vi "AlliGator Get Control Notebook String.vi"(8 "error in (no error)":errorcluster, 9 "Value":variant, 11 "Control Label":string) -> (0 "error out":errorcluster, 3 "Notebook String":string)   [LabVIEW 2021, in "AlliGator Settings.lvlib"]
doc: "Formats the input <B>Value</B> of the control whose <B>Control Label</b> is provided into a string.\n\nA special case is needed when units are involved, otherwise the default case should be able to handle all other cases."
uses:
  AlliGator Settings.lvlib
  Graphs/XY Graph/XY Graph Plot Shift Method.ctl
  AlliGator Settings List.ctl
  Decay Analysis/Decay Preprocessing/AlliGator Baseline Subtraction Method.ctl
  Phasor/Phasor Calibration Type.ctl
  Phasor Calibration/AlliGator Calibration Map Algorithm.ctl
  Phasor/Phasor Explorer Decay Parameters.ctl
  Phasor/Phasor IRF Model.ctl
  Graphs/XY Graph/XY Graph Plot Shift Parameters.ctl
  AlliGator Define Gates to.ctl
  Phasor/Phasor Explorer Display Parameters.ctl
  Phasor/Phasor Type of Series.ctl
  Fits/IRF(X)PSED/Decay Fit Parameters & Derived Quantities List v2.ctl
  Decay Analysis/Decay Fit/AlliGator Decay Fit Parameter Constraints 2.ctl
  Fits/IRF(X)PSED/Decay Fit Parameters In List.ctl
  Phasor/Phasor Explorer Gate Parameters.ctl
  Phasor/Phasor Gate Type.ctl
  Phasor/Phasor Type of User-defined Function.ctl
  AlliGator Gate Arithmetic.ctl
  AlliGator Gates to Keep.ctl
  Fits/IRF(X)PSED/MLE Baseline Offset Type.ctl
  AlliGator Background Subtraction Parameters.ctl
  SwissSPAD/SwissSPAD Live_Image Display Options.ctl
  Phasor/Phasor Ratio Type.ctl
  AlliGator High Count Pixels Rejection Options.ctl
  Fits/IRF(X)PSED/IRF(X)PSED Extraction Options.ctl
  Fits/IRF(X)PSED/Fourier Series Smoothing Option.ctl
  Fits/IRF(X)PSED/Fourier Series Truncation.ctl
  Fits/IRF(X)PSED/IRF Extraction Method.ctl
  Arrays/Kernel Type.ctl
  AlliGator Low Count Pixels Rejection Options.ctl
  Phasor/Phasor Explorer Phasor Parameters.ctl
  Phasor/Phasor Calculation Type.ctl
  Phasor/Phasor SEPL Type.ctl
  Phasor Plot/AlliGator Phasor Plot Size.ctl
  Phasor Ratio/AlliGator Phasor Ratio Color-Coded Quantity.ctl
  Phasor/Pseudo UC Additional Parameters.ctl
  AlliGator Python Settings.ctl
  Image/Image Save File Format.ctl
  Fits/Square Pulse/Square Pulse Options.ctl
  Fits/Square Pulse/Square Pulse Levels Type.ctl
  Graphs/XY Graph/XY Graph Plot Data.ctl
  Math/Advanced Signal Processing Toolkit/Wavelet Analysis Options.ctl
  Variant/Variant to Data/Variant to U32.vi
  Variant/Variant to Data/Variant to I32.vi
  Variant/Variant to Data/Variant to String.vi
  Variant/Variant to Data/Variant to Boolean.vi
  Variant/Variant to Data/Variant to DBL.vi
  Variant/Variant to Data/Variant to Path.vi
  Variant/Variant to Data/Variant to [String].vi
  Variant/Variant to Data/Variant to U16.vi
  Variant/Variant to Data/Variant to [DBL].vi
  Variant/Variant to Data/Variant to Data.lvlib
  Phasor Plot/AlliGator Phasor Plot.lvlib
  Graphs/XY Graph/XY Graph Add-Ons.lvlib
  Image/Image.lvlib
  Decay Analysis/Decay Preprocessing/AlliGator Decay Preprocessing.lvlib
  Fits/Fits.lvlib
  Decay Analysis/Decay Fit/AlliGator Decay Fit.lvlib
  Phasor/Phasor.lvlib
  Strings/Strings.lvlib
  Arrays/Arrays.lvlib
  Math/Math.lvlib
  Phasor/Phasor Explorer.lvlib
  Phasor Ratio/AlliGator Phasor Ratio.lvlib
  Phasor Calibration/AlliGator Phasor Calibration.lvlib
  SwissSPAD/SwissSPAD Live.lvlib
  Variant/Variant.lvlib
panel:
  in  "Type":T1
  # "see the AlliGator License on the block diagram (Ctrl+E or Window:Show Block Diagram)"
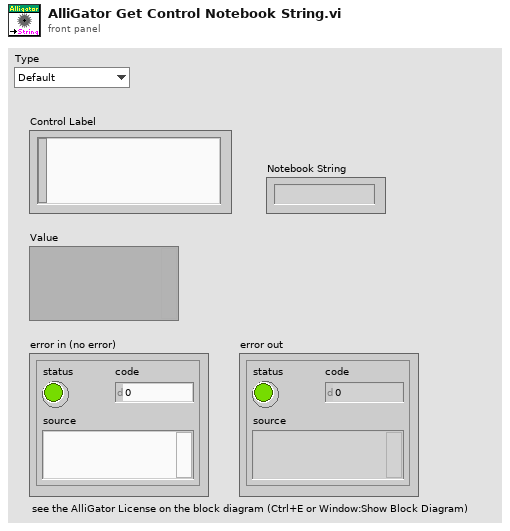
[diagram p1: front panel]
types:
  T1 = typedef "XY Graph Add-Ons.lvlib/XY Graph Plot Shift Method.ctl" = enum16{"Default", "CFD", "Threshold", "Cross-Correlation"}
  T2 = typedef "AlliGator Settings.lvlib/AlliGator Settings List.ctl" = enum16{"GUI:Visible Settings Tab", "GUI:Last Run Version", "Source Image:Use Image Histogram for Contrast", "Source Image:Low Count Pixels Rejection Options", "Source Image:High Count Pixels Rejection Options", "Source Image:Use Image Brightness", "Source Image:Blend Overlay with Image Background", "Source Image:Use Fixed ROI Diameter", "Source Image:ROI Diameter", "Source Image:ROI Center Color", "Source Image:Peak Threshold", "Source Image:Intensity Threshold", "Source Image:Image Binning Options", "Source Image:Image Smoothing Options", "Source Image:Image Histogram Active", "Source Image:Invert Binary Mask", "Source Image:Hot Pixel Removal", "Source Image:Overlay Analyzed ROI Center", "Source Image:Auto-Adjust Contrast", "Source Image:Histogram Lower Percentile", "Source Image:Histogram Upper Percentile", "Source Image:Save Source Image", "Source Image:Scale Bar Options", "Source Image:Image Resolution (Pixel Size)", "Source Image:Flatfield Correction", "Source Image:Show Dead Left Columns Correction", "Source Image:Dead Left Columns Correction", "Source Image:Image Pre-Processing Operations Order", "Source Image:Overlay ROI Median", "Source Image:Median Overlay Color", "Data Information:Gate Width", "Data Information:Nanotime Gate Separation", "Data Information:Macrotime Gate Separation", "Data Information:Gate Step", "Data Information:# Gates", "Data Information:Gate Image Exposure", "Data Information:Gate Image Integration", "Data Information:Gates to Skip", "Data Information:Gates to Keep", "Data Information:Define Gates to", "Data Information:Channel Name", "Data Information:Available Channel Names", "Data Information:Channel Arithmetic", "Data Information:Background File Subtraction", "Data Information:Background File", "Data Information:Background Scaling Factor", "Data Information:Background Pile-up Correction", "Data Information:Background Pixel Well Capacity", "Data Information:Laser Period", "Data Information:SYNC Period", "Data Information:Pile-up Correction", "Data Information:Pixel Well Capacity", "Data Information:Dataset Scaling Factor", "Fluorescence Decay_Decay Pre-Processing:Reverse Gates", "Fluorescence Decay_Decay Pre-Processing:Verbose Decay Pre-Processing", "Fluorescence Decay_Decay Pre-Processing:Use Decay Pre-Processing", "Fluorescence Decay_Decay Pre-Processing:Background Subtraction", "Fluorescence Decay_Decay Pre-Processing:Background Definition Range", "Fluorescence Decay_Decay Pre-Processing:Baseline Subtraction Method", "Fluorescence Decay_Decay Pre-Processing:Decay Pre-Processing Operations Order", "Fluorescence Decay_Decay Pre-Processing:Smoothing Parameter", "Fluorescence Decay_Decay Pre-Processing:Shift Decay", "Fluorescence Decay_Decay Pre-Processing:Decay Shift Parameters", "Fluorescence Decay_Decay Pre-Processing:Fold Decay", "Fluorescence Decay_Decay Pre-Processing:# Folds", "Fluorescence Decay_Decay Pre-Processing:1-Normalize Decay", "Fluorescence Decay_Decay Pre-Processing:[0-1]-Normalize Decay", "Fluorescence Decay_Decay Pre-Processing:Smoothen Decay", "Fluorescence Decay_Decay Pre-Processing:Extrapolate Decay", "Fluorescence Decay_Decay Pre-Processing:Use Periodicity", "Fluorescence Decay_Decay Pre-Processing:Use Cursors", "Fluorescence Decay_Decay Pre-Processing:Tail Fraction", "Fluorescence Decay_Decay Pre-Processing:Head Fraction", "Fluorescence Decay_Decay Pre-Processing:Additional Points", "Fluorescence Decay_Decay Pre-Processing:Straighten Decay", "Fluorescence Decay_Decay Pre-Processing:Constant Background", "Fluorescence Decay_Decay Pre-Processing:Pixel-Normalize Decay", "Fluorescence Decay_Advanced Analysis:Extract IRF instead of Decay", "Fluorescence Decay_Advanced Analysis:IRF Extraction Options", "Fluorescence Decay_Advanced Analysis:IRF Optimization Options", "Fluorescence Decay_Advanced Analysis:Square Pulse Options", "Fluorescence Decay_Advanced Analysis:IRF Order", "Fluorescence Decay_Advanced Analysis:IRF Time Constants", "Fluorescence Decay_Advanced Analysis:Wavelet Analysis Options", "Fluorescence Decay_Advanced Analysis:Average Lifetime Options", "Fluorescence Decay_Fit Options:Fit Options", "Fluorescence Decay_Fit Options:Use Legacy Fitting Approach", "Fluorescence Decay_Fit Options:Use Data Information Laser Period", "Fluorescence Decay_Fit Parameters:Displayed Fit Parameters", "Fluorescence Decay_Fit Parameters:Fit Parameter Constraints", "Fluorescence Decay_Fit Parameters:Export Tabulated Results", "Fluorescence Decay_Fit Parameters:MLE Baseline Offset Type", "Fluorescence Decay_Fit Parameters:MLE Baseline Offset", "Fluorescence Decay_Fit Parameters:Guess Parameter Names", "Fluorescence Decay_Fit Parameters:Guess Parameter Values", "Fluorescence Decay_Fit Parameters:Guess Parameters Options", "Fluorescence Decay_Fit Parameters:Optimal Offset Selection Criterion", "Fluorescence Decay_Styles:Show Last Decay Only", "Fluorescence Decay_Styles:Decay Graph Color Array", "Fluorescence Decay:Decay Graph Active", "Fluorescence Decay Statistics:Min Peak Value", "Fluorescence Decay Statistics:Reject Low Decay Peak Pixels", "Fluorescence Decay Statistics:Reject High Decay Peak Pixels", "Fluorescence Decay Statistics:Max Peak Value", "Time Traces:Use File Timestamp", "Time Traces:Time Step", "Time Traces:Use Intensity Correction File", "Time Traces:Intensity Correction File", "Phasor Plot:Phasor Plot Smoothing Options", "Phasor Plot:Phasor Plot Size", "Phasor Plot:Phasor Plot Graphics Options", "Phasor Plot:Cumulative Phasor Plot", "Phasor Plot:Use Phasor Brightness", "Phasor Plot:Blend Overlay with Phasor Background", "Phasor Plot:Save Phasor Plot", "Phasor Plot:Show References", "Phasor Plot:Phasor Ratio Decay Range", "Phasor Plot:Exponential Fading", "Phasor Plot:Phasor Ratio Reference Colors", "Phasor Plot:Reference Radius", "Phasor Plot:Show Color Map Vertices", "Phasor Plot:Phasor Plot Active", "Phasor Plot:Phasor Ratio Color Map Type", "Phasor Plot:Phasor Ratio Color Map", "Phasor Plot:Phasor Ratio Display Range", "Phasor Plot:Selected Image ROI(s)", "Phasor Plot:All Image ROIs", "Phasor Plot:Selected Phasor Plot ROI(s)", "Phasor Plot:All Phasor Plot ROIs", "Phasor Plot:Phasor Ratio Color-Coded Quantity", "Phasor Plot:Store Phasor Harmonics", "Phasor Plot:Draw Reference Segment", "Phasor Plot:User-Defined Quantity", "Phasor Plot:Color Scale High Color", "Phasor Plot:Color Scale Low Color", "Phasor Graph:Phasor Frequency", "Phasor Graph:Phasor Ratio Type", "Phasor Graph:Pixel-level Phasor Computation", "Phasor Graph:Save Phasor Graph", "Phasor Graph:Phasor Graph Active", "Phasor Graph:Phasor SDV Options", "Phasor Calibration:Use Backup Calibration if needed", "Phasor Graph:Define Shortest Lifetime as", "Phasor Calibration:Backup Calibration Type", "Phasor Calibration:Calibration Type", "Phasor Calibration:Calibration Lifetime", "Phasor Calibration:Calibration Map Algorithm", "Single-Exponential Phasor Locus (SEPL):Gate Parameters", "Single-Exponential Phasor Locus (SEPL):User-defined Gate", "Single-Exponential Phasor Locus (SEPL):User-defined IRF", "Single-Exponential Phasor Locus (SEPL):Phasor Parameters", "Single-Exponential Phasor Locus (SEPL):Decay & IRF Parameters", "Single-Exponential Phasor Locus (SEPL):Display Parameters", "Lifetime Analysis:Decay Analysis Parameters", "Lifetime Analysis:Lifetime Map Active", "Plugins:Python Settings", "Miscellaneous:Verbose Mode", "Miscellaneous:Beep after Script", "Miscellaneous:Saved Image File Format", "Miscellaneous:Exported Gate Image Settings", "Miscellaneous:Include Loading in Timing", "Miscellaneous:Verbose Settings Mode", "Miscellaneous:Histogram Options", "Miscellaneous:Beep on Error", "Miscellaneous:# Logical Processors Used", "Miscellaneous:ROI Description Max Characters", "Miscellaneous:Verbose Error Mode", "Miscellaneous:Transparent Mask Color"}
  T3 = cluster{"Min Gate":dbl[unit], "Max Gate":dbl[unit]}
  T4 = enum16{"Single Calibration", "Nearest Valid Calibration"}
  T5 = typedef "AlliGator Decay Preprocessing.lvlib/AlliGator Baseline Subtraction Method.ctl" = enum16{"Mean", "Min", "Square Gated Single-Exponential", "File", "Constant"}
  T6 = typedef "Phasor.lvlib/Phasor Calibration Type.ctl" = enum16{"None", "Single Phasor", "Phasor Series", "Phasor Map"}
  T7 = typedef "AlliGator Phasor Calibration.lvlib/AlliGator Calibration Map Algorithm.ctl" = enum16{"Simple Search", "Min Distance"}
  T8 = typedef "Phasor Explorer.lvlib/Phasor Explorer Decay Parameters.ctl" = cluster{"Lifetime":dbl[unit], "IRF Offset":dbl[unit], "IRF Period":dbl[unit], "Normalized Decays":bool, "IRF Model":T9, "IRF Parameter 1":dbl[unit]}
  T9 = typedef "Phasor.lvlib/Phasor IRF Model.ctl" = enum16{"Dirac", "Exponential"}
  T10 = typedef "XY Graph Add-Ons.lvlib/XY Graph Plot Shift Parameters.ctl" = cluster{"Type":T1, "Shift":dbl[unit], "Threshold":dbl, "Rotate":bool}
  T11 = typedef "AlliGator Settings.lvlib/AlliGator Define Gates to.ctl" = enum32{"Skip", "Keep"}
  T12 = typedef "Phasor Explorer.lvlib/Phasor Explorer Display Parameters.ctl" = cluster{"# Points":i32, "Ramp Type":enum16{"Linear", "Logarithmic"}, "Type of Series":T13, "Min tau":dbl[unit], "Max tau":dbl[unit], "Include 0":bool, "Include Infinity":bool}
  T13 = typedef "Phasor.lvlib/Phasor Type of Series.ctl" = enum16{"1-Exp Decays", "Linear Combination of 1-Exp"}
  T14 = typedef "AlliGator Decay Fit.lvlib/AlliGator Decay Fit Parameter Constraints 2.ctl" = cluster{"Fit Parameter":T15, "Min Value":dbl, "Max Value":dbl, "Global":bool, "Used":bool}
  T15 = typedef "Fits.lvlib/Decay Fit Parameters In List.ctl" = enum16{"Offset", "Baseline", "A_1", "tau_1", "A_2", "tau_2"}
  T16 = typedef "Phasor Explorer.lvlib/Phasor Explorer Gate Parameters.ctl" = cluster{"First Gate Start":dbl[unit], "Use Gate Center":bool, "Gate Width":dbl[unit], "Gate Step":dbl[unit], "# Gates":dbl, "Gate Type":T17, "Edge Width":dbl[unit], "Top Slope":dbl[unit], "Reversed Sawtooth?":bool, "Analytical Computation":bool, "Integration":enum32{"Item 0", "Item 1"}, "Tolerance":dbl, "# Steps":dbl, "Type of User-defined Function":T18, "Use Gate Step":bool}
  T17 = typedef "Phasor.lvlib/Phasor Gate Type.ctl" = enum16{"Square", "Finite Edge Square", "Finite Edge, Tilted Top Square", "Triangle", "Sawtooth", "User-defined"}
  T18 = typedef "Phasor.lvlib/Phasor Type of User-defined Function.ctl" = enum16{"Gate", "IRF"}
  T19 = typedef "AlliGator Settings.lvlib/AlliGator Gate Arithmetic.ctl" = enum16{"None", "INT-G2", "G2/INT*<INT>", "(1 - G2/INT)*<INT>"}
  T20 = typedef "AlliGator Settings.lvlib/AlliGator Gates to Keep.ctl" = cluster{"First":u32, "Last":u32}
  T21 = typedef "Fits.lvlib/MLE Baseline Offset Type.ctl" = enum32{"Absolute", "Percentage"}
  T22 = typedef "AlliGator Settings.lvlib/AlliGator Background Subtraction Parameters.ctl" = cluster{"Start":u32, "End":u32}
  T23 = typedef "SwissSPAD Live.lvlib/SwissSPAD Live_Image Display Options.ctl" = cluster{"Remove Screamers":bool, "Delta":sgl, "Equalize Histogram":bool, "Percentile":sgl, "Hot Pixel Mask Image":path, "Use Hot Pixel Mask":bool}
  T24 = typedef "Phasor.lvlib/Phasor Ratio Type.ctl" = enum32{"Intensity-weighted", "Amplitude-weighted"}
  T25 = typedef "AlliGator Settings.lvlib/AlliGator High Count Pixels Rejection Options.ctl" = cluster{"Background High Threshold Factor":dbl, "Fixed High Background Threshold":dbl, "Reject High Count Pixels":bool, "High Percentile":dbl}
  T26 = typedef "Fits.lvlib/IRF(X)PSED Extraction Options.ctl" = cluster{"Time Constant for IRF Extraction":dbl[unit], "IRF Order":i32, "Fourier Series Smoothing":T27, "Noise Threshold":dbl, "Smoothing Width":dbl, "Fourier Series Truncation":T28, "Truncation Order":i32, "Save Power Spectrum":bool, "Smoothing":bool, "Smoothing Parameter":dbl, "Smoothing Order":u32, "Method":T29}
  T27 = typedef "Fits.lvlib/Fourier Series Smoothing Option.ctl" = enum16{"None", "Lanczos Factors", "Fejer Summation"}
  T28 = typedef "Fits.lvlib/Fourier Series Truncation.ctl" = enum16{"Automatic", "Fixed"}
  T29 = typedef "Fits.lvlib/IRF Extraction Method.ctl" = enum16{"Direct", "Topless", "Toeplitz"}
  T30 = typedef "Arrays.lvlib/Kernel Type.ctl" = enum16{"Uniform", "Bilinear", "Gaussian"}
  T31 = typedef "AlliGator Settings.lvlib/AlliGator Low Count Pixels Rejection Options.ctl" = cluster{"Background Low Threshold Factor":dbl, "Fixed Low Background Threshold":dbl, "Reject Low Count Pixels":bool, "Low Percentile":dbl}
  T32 = typedef "Phasor Explorer.lvlib/Phasor Explorer Phasor Parameters.ctl" = cluster{"Harmonic Frequency":dbl[unit], "Use f* = 1/D Frequency":bool, "Calibrated Phasor":bool, "Calibration Lifetime":dbl[unit], "Phasor Calculation":T33, "SEPL Type":T34, "# Gates":dbl, "Square Gate Width":dbl[unit], "Show Ticks":bool}
  T33 = typedef "Phasor.lvlib/Phasor Calculation Type.ctl" = enum16{"Direct Sum", "Analytical Formula"}
  T34 = typedef "Phasor.lvlib/Phasor SEPL Type.ctl" = enum16{"UC", "L_N", "L_N[W]", "L_X"}
  T35 = typedef "AlliGator Phasor Plot.lvlib/AlliGator Phasor Plot Size.ctl" = cluster{"H":i32, "V":i32, "Margin":dbl}
  T36 = enum32{"Interpolate Reference Colors", "Use Custom Map"}
  T37 = typedef "AlliGator Phasor Ratio.lvlib/AlliGator Phasor Ratio Color-Coded Quantity.ctl" = enum16{"Phasor Ratio (f1 or a1)", "Average Lifetime (<tau>_i or <tau>_a))", "User-Defined Quantity"}
  T38 = cluster{"Reference 1":u32, "Reference 2":u32, "Boundary":u32}
  T39 = typedef "Phasor.lvlib/Pseudo UC Additional Parameters.ctl" = cluster{"Laser Period":dbl[unit], "Decay Offset":dbl[unit]}
  T40 = typedef "AlliGator Settings.lvlib/AlliGator Python Settings.ctl" = cluster{"Python Version":string, "Use PATH definition":bool, "Python.exe Path":path, "Include Example Plugins":bool}
  T41 = typedef "Image.lvlib/Image Save File Format.ctl" = enum16{"PNG", "JPEG", "BMP"}
  T42 = typedef "Fits.lvlib/Square Pulse Options.ctl" = cluster{"Method":T43, "# Bins":i32, "Threshold %":dbl, "Center on Midpoint":bool, "Smoothen Plot":bool}
  T43 = typedef "Fits.lvlib/Square Pulse Levels Type.ctl" = enum16{"Mode", "Mean"}
  T44 = typedef "XY Graph Add-Ons.lvlib/XY Graph Plot Data.ctl" = cluster{"X Array":dbl[], "Y Array":dbl[]}
  T45 = typedef "Math.lvlib/Wavelet Analysis Options.ctl" = cluster{"Wavelet":enum16{"db02", "db03", "db04", "db05", "db06", "db07", "db08", "db09", "db10", "db11", "db12", "db13", "db14", "Haar", "bior1_3", "bior1_5", "bior2_2", "bior2_4", "bior2_6", "bior2_8", "bior3_1", "bior3_3", "bior3_5", "bior3_7", "bior3_9", "bior4_4 (FBI)", "bior5_5", "bior6_8", "coif1", "coif2", "coif3", "coif4", "coif5", "sym2", "sym3", "sym4", "sym5", "sym6", "sym7", "sym8"}, "Option for Approximate Coefficients":enum16{"None", "Threshold", "Detrend"}, "# Levels":i32, "Threshold Settings":cluster{"Thresholding Rule":enum16{"SURE", "Hybrid", "Universal", "Minimax"}, "Rescaling Method":enum16{"One", "Single level", "Multiple levels"}, "Soft Threshold?":bool}, "Wavelet Transform Type":enum16{"Discrete", "Undecimated"}}
  T46 = typedef "Fits.lvlib/Decay Fit Parameters & Derived Quantities List v2.ctl" = enum16{"Offset", "Baseline", "A_1", "tau_1", "A_2", "tau_2", "<tau>_a", "f1_a", "f2_a", "<tau>_i", "f1_i", "f2_i", "-", "R^2", "Chi^2"}
  T47 = enum16{"db02", "db03", "db04", "db05", "db06", "db07", "db08", "db09", "db10", "db11", "db12", "db13", "db14", "Haar", "bior1_3", "bior1_5", "bior2_2", "bior2_4", "bior2_6", "bior2_8", "bior3_1", "bior3_3", "bior3_5", "bior3_7", "bior3_9", "bior4_4 (FBI)", "bior5_5", "bior6_8", "coif1", "coif2", "coif3", "coif4", "coif5", "sym2", "sym3", "sym4", "sym5", "sym6", "sym7", "sym8"}
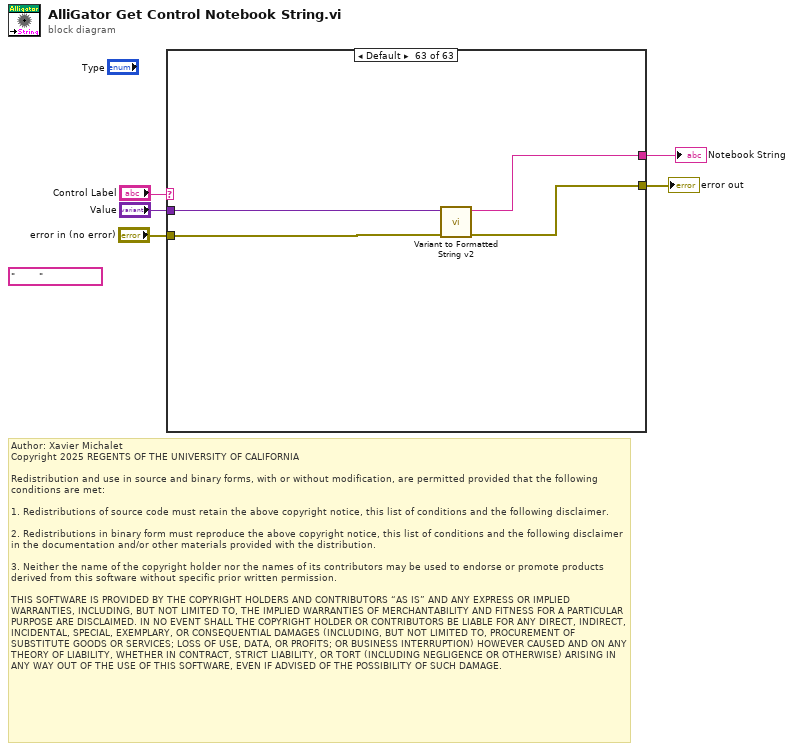
[diagram p0: block diagram]
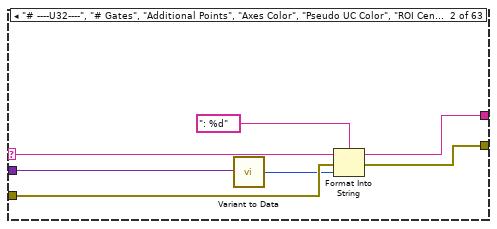
[diagram p3: hidden frame]
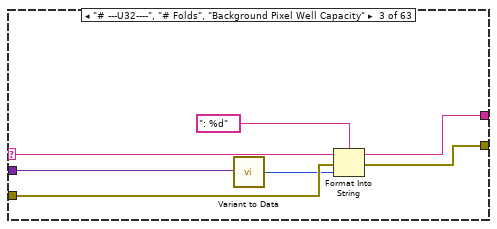
[diagram p4: hidden frame]
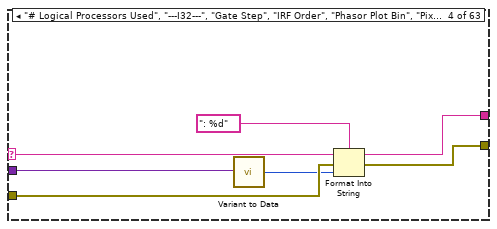
[diagram p5: hidden frame]
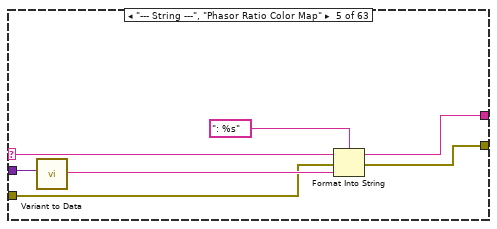
[diagram p6: hidden frame]
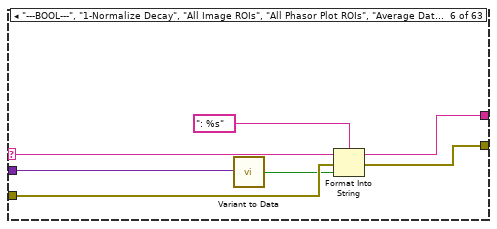
[diagram p7: hidden frame]
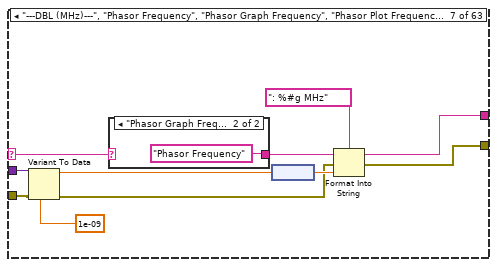
[diagram p8: hidden frame]
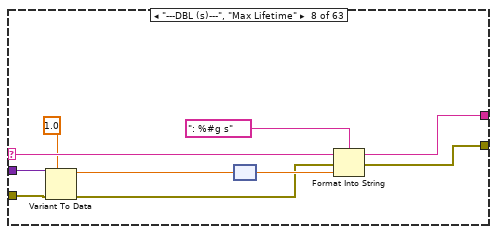
[diagram p10: hidden frame]
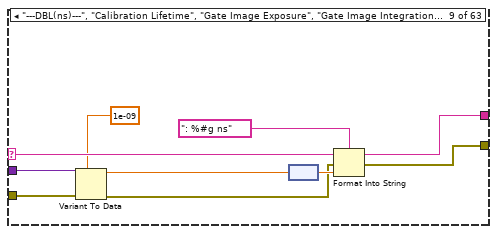
[diagram p11: hidden frame]
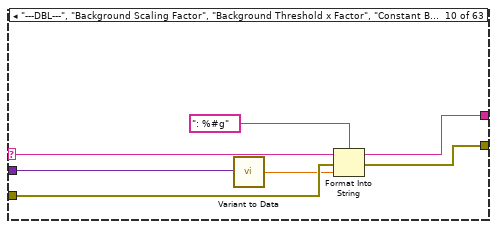
[diagram p12: hidden frame]
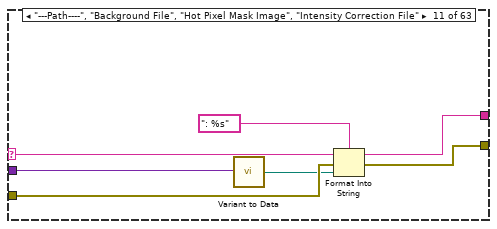
[diagram p13: hidden frame]
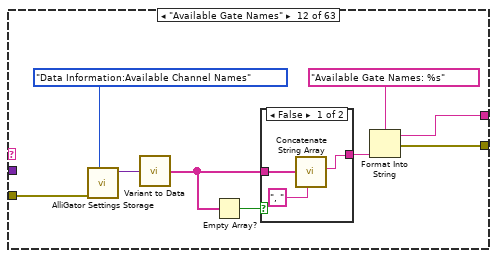
[diagram p14: hidden frame]
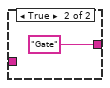
[diagram p15: hidden frame]
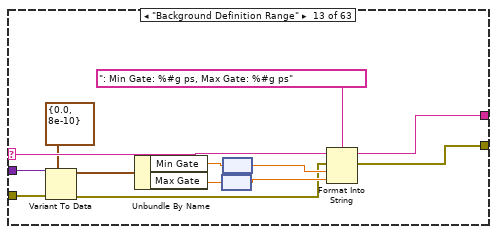
[diagram p16: hidden frame]
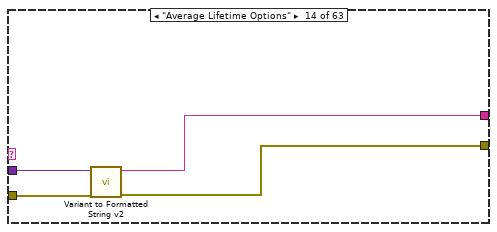
[diagram p17: hidden frame]
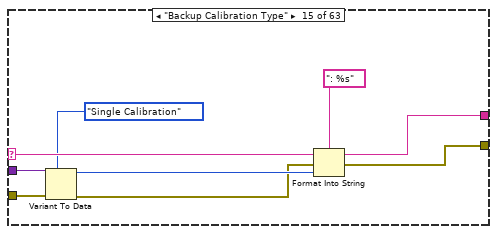
[diagram p18: hidden frame]
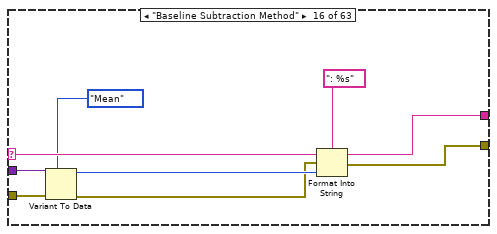
[diagram p19: hidden frame]
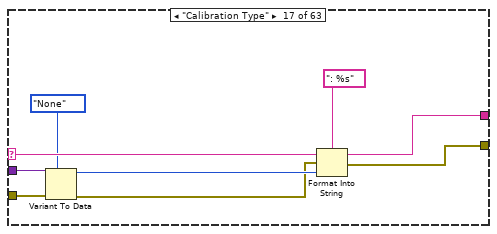
[diagram p20: hidden frame]
diagram:
  (unwired) "        " ("Separator (TAB)")
  # "Author: Xavier Michalet\nCopyright 2025 REGENTS OF THE UNIVERSITY OF CALIFORNIA\n\nRedistribution and use in source and binary forms, with or without modification, are permitted provided that the following conditions are met:\n\n1. Redistributions of source code must retain the above copyright notice, this list of conditions and the following disclaimer.\n\n2. Redistributions in binary form must reproduce the above copyright notice, this list of conditions and the following disclaimer in the documentation and/or other materials provided with the distribution.\n\n3. Neither the name of the copyright holder nor the names of its contributors may be used to endorse or promote products derived from this software without specific prior written permission.\n\nTHIS SOFTWARE IS PROVIDED BY THE COPYRIGHT HOLDERS AND CONTRIBUTORS “AS IS” AND ANY EXPRESS OR IMPLIED WARRANTIES, INCLUDING, BUT NOT LIMITED TO, THE IMPLIED WARRANTIES OF MERCHANTABILITY AND FITNESS FOR A PARTICULAR PURPOSE ARE DISCLAIMED. IN NO EVENT SHALL THE COPYRIGHT HOLDER OR CONTRIBUTORS BE LIABLE FOR ANY DIRECT, INDIRECT, INCIDENTAL, SPECIAL, EXEMPLARY, OR CONSEQUENTIAL DAMAGES (INCLUDING, BUT NOT LIMITED TO, PROCUREMENT OF SUBSTITUTE GOODS OR SERVICES; LOSS OF USE, DATA, OR PROFITS; OR BUSINESS INTERRUPTION) HOWEVER CAUSED AND ON ANY THEORY OF LIABILITY, WHETHER IN CONTRACT, STRICT LIABILITY, OR TORT (INCLUDING NEGLIGENCE OR OTHERWISE) ARISING IN ANY WAY OUT OF THE USE OF THIS SOFTWARE, EVEN IF ADVISED OF THE POSSIBILITY OF SUCH DAMAGE."
  n1 = case shown="Default" "Control Label" {
    selector: "Control Label" -> [_ w13 w20 w27 w34 w41 w45 w64 w74 w81 w88 _ w114 _ w127 w136 w145 w154 _ w176 w200 _ _ _ w246 _ w269 _ _ w314 w329 w338 w349 _ w366 w377 w388 w403 w417 w459 _ _ w473 w486 w495 w502 _ w524 w536 w540 w546 w565 w577 w590 w601 w610 w619 w625 _ _ w648 w679 _]
    tunnel: "error in (no error)" -> [w6 w12 w19 w26 w28 w40 w43 w56 w66 w80 w87 w94 w103 w117 w120 w129 w139 w148 w160 w164 w202 w219 w230 w242 w250 w264 w271 w296 w308 w317 w320 w333 w340 w352 w361 w374 w390 w393 w405 w453 w462 w464 w466 w475 w488 w498 w512 w515 w526 w544 w549 w557 w567 w579 w595 w604 w612 w627 w633 w637 w656 w671 w681]
    tunnel: "Value" -> [_ w10 w17 w24 w30 w38 w49 w60 w70 w78 w85 _ w110 w118 w123 w132 w141 w150 w161 w172 w203 w220 w231 w243 w251 w265 w272 w297 w309 w318 w325 w334 w345 w354 w362 w375 w389 w399 w414 w456 w463 _ w469 w482 _ w506 w513 w520 w532 w545 w551 w561 w573 w587 w598 w607 w615 w628 w635 w640 w655 w676 w680]
    tunnel: [_ w8 w15 w22 w32 w36 w51 w62 w72 w76 w83 w96 w112 w116 w125 w134 w143 w152 w157 w174 w199 w222 w233 w239 w248 w263 w274 w299 w304 w311 w327 w336 w347 w356 w364 w376 w387 w401 w416 w458 w460 _ w471 w484 w496 w499 w509 w522 w534 w541 w553 w563 w575 w589 w600 w609 w617 w622 w630 w642 w650 w678 w683] -> w3
    tunnel: [w6 w7 w14 w21 w31 w35 w50 w61 w71 w75 w82 w95 w111 w115 w124 w133 w142 w151 w156 w173 w198 w221 w232 w238 w247 w262 w273 w298 w303 w312 w326 w335 w346 w355 w363 w373 w390 w400 w415 w457 w461 w464 w470 w483 w497 w505 w508 w521 w533 w542 w552 w562 w574 w588 w599 w608 w616 w620 w629 w641 w649 w677 w682] -> w4
    frame "" {
    }
    frame "# ----U32----", "# Gates", "Additional Points", "Axes Color", "Pseudo UC Color", "ROI Center Color", "UC Color" {
      n2 = call-poly "Variant to Data.vi"("Variant"=w10) -> ("Value"=w9:u32)  [unwired: 8 in]
      n3 = Format Into String(format string=": %d", initial string=w13, error in=w12, w9) -> (resulting string=w8:string, error out=w7:errorcluster)
    }
    frame "# ---U32----", "# Folds", "Background Pixel Well Capacity" {
      n4 = call-poly "Variant to Data.vi"("Variant"=w17) -> ("Value"=w16:u32)  [unwired: 8 in]
      n5 = Format Into String(format string=": %d", initial string=w20, error in=w19, w16) -> (resulting string=w15:string, error out=w14:errorcluster)
    }
    frame "# Logical Processors Used", "---I32---", "Gate Step", "IRF Order", "Phasor Plot Bin", "Pixel Well Capacity", "ROI Diameter", "Reference Radius" {
      n6 = call-poly "Variant to Data.vi"("Variant"=w24) -> ("Value"=w23:i32)  [unwired: 8 in]
      n7 = Format Into String(format string=": %d", initial string=w27, error in=w26, w23) -> (resulting string=w22:string, error out=w21:errorcluster)
    }
    frame "--- String ---", "Phasor Ratio Color Map" {
      n8 = call-poly "Variant to Data.vi"("Variant"=w30) -> ("String"=w29:string)  [unwired: 8 in]
      n9 = Format Into String(format string=": %s", initial string=w34, error in=w28, w29) -> (resulting string=w32:string, error out=w31:errorcluster)
    }
    frame "---BOOL---", "1-Normalize Decay", "All Image ROIs", "All Phasor Plot ROIs", "Average Dataset Sum", "Background File Subtraction", "Background Pile-up Correction", "Background Subtraction", "Beep after Script", "Beep on Error", "Blend Overlay with Image Background", "Blend Overlay with Phasor Background", "Compute <INT> + INT - 2 G2", "Cumulative Phasor Plot", "Decay Graph Active", "Draw Reference Segment", "Exponential Fading", "Export Tabulated Results", "Extract IRF instead of Decay", "Extrapolate Decay", "Fold Decay", "Image Histogram Active", "Include Loading in Timing", "Invert Binary Mask", "Overlay Analyzed ROI Center", "Phasor Graph Active", "Phasor Plot Active", "Pile-up Correction", "Pixel-Normalize Decay", "Pixel-level Phasor Computation", "Reject High Count Pixels", "Reject High Decay Peak Pixels", "Reject Low Count Pixels", "Reject Low Decay Peak Pixels", "Reverse Gates", "Save Image", "Save Phasor Graph", "Save Phasor Plot", "Save Source Image", "Selected Image ROI(s)", "Selected Phasor Plot ROI(s)", "Shift Decay", "Show Color Map Vertices", "Show Last Decay Only", "Show Line", "Show Pseudo UC", "Show References", "Show SEPL Plot Ticks", "Show UC", "Show UC Plot Ticks", "Show UC Ticks", "Smoothen Decay", "Store Phasor Harmonics", "Straighten Decay", "Use Backup Calibration if needed", "Use Calibration Phasor", "Use Calibration Phasor Map", "Use Calibration Phasor Series", "Use Cursors", "Use Decay Pre-Processing", "Use File Timestamp", "Use Fixed ROI Diameter", "Use Gate Center", "Use Guess Parameters", "Use Image Brightness", "Use Image Histogram for Contrast", "Use Intensity Correction File", "Use Last Fitted Parameters", "Use Legacy Fitting Approach", "Use Periodicity", "Use Phasor Brightness", "Use Phasor Calibration Map", "Use Phasor Plot Binning", "Use Single Phasor Calibration", "Verbose Decay Pre-Processing", "Verbose Error Mode", "Verbose Mode", "Verbose Settings Mode", "[0-1]-Normalize Decay" {
      n10 = call-poly "Variant to Data.vi"("Variant"=w38) -> ("Value"=w37:bool)  [unwired: 8 in]
      n11 = Format Into String(format string=": %s", initial string=w41, error in=w40, w37) -> (resulting string=w36:string, error out=w35:errorcluster)
    }
    frame "---DBL (MHz)---", "Phasor Frequency", "Phasor Graph Frequency", "Phasor Plot Frequency" {
      n12 = Variant To Data(error in=w43, type=dbl[unit] 1e-09 ("Time Constant for IRF Extraction"), Variant=w49) -> (data=w48:dbl[unit], error out=w42:errorcluster)
      n13 = case shown="\"Phasor Graph Frequency\", \"Phasor Plot Frequency\"" w45 {
        selector: w45 -> [w53 _]
        tunnel: [w53 "Phasor Frequency"] -> w44
        frame "False", Default {
        }
        frame "Phasor Graph Frequency", "Phasor Plot Frequency" {
        }
      }
      n14 = node(w48) -> (w46:dbl)
      n15 = Format Into String(format string=": %#g MHz", initial string=w44, error in=w42, w46) -> (resulting string=w51:string, error out=w50:errorcluster)
    }
    frame "---DBL (s)---", "Max Lifetime" {
      n16 = Variant To Data(error in=w56, type=dbl[unit] 1.0 ("Time Constant for IRF Extraction"), Variant=w60) -> (data=w59:dbl[unit], error out=w55:errorcluster)
      n17 = node(w59) -> (w57:dbl)
      n18 = Format Into String(format string=": %#g s", initial string=w64, error in=w55, w57) -> (resulting string=w62:string, error out=w61:errorcluster)
    }
    frame "---DBL(ns)---", "Calibration Lifetime", "Gate Image Exposure", "Gate Image Integration", "Gate Separation", "Gate Width", "IRF Period", "Laser Period", "Period", "SYNC Period", "Shift", "Time Constant for IRF Extraction", "Time Step" {
      n19 = Variant To Data(error in=w66, type=dbl[unit] 1e-09 ("Time Constant for IRF Extraction"), Variant=w70) -> (data=w69:dbl[unit], error out=w65:errorcluster)
      n20 = node(w69) -> (w67:dbl)
      n21 = Format Into String(format string=": %#g ns", initial string=w74, error in=w65, w67) -> (resulting string=w72:string, error out=w71:errorcluster)
    }
    frame "---DBL---", "Background Scaling Factor", "Background Threshold x Factor", "Constant Background", "Dataset Scaling Factor", "Fixed Background Threshold", "Fixed Peak Threshold", "Head Fraction", "Intensity Threshold", "MLE Baseline Offset", "Max Peak Value", "Min Peak Value", "Peak Threshold", "Peak Threshold x Factor", "Phasor Ratio Decay Range", "Smoothing Parameter", "Tail Fraction", "Threshold" {
      n22 = call-poly "Variant to Data.vi"("Variant"=w78) -> ("Value"=w77:dbl)  [unwired: 8 in]
      n23 = Format Into String(format string=": %#g", initial string=w81, error in=w80, w77) -> (resulting string=w76:string, error out=w75:errorcluster)
    }
    frame "---Path----", "Background File", "Hot Pixel Mask Image", "Intensity Correction File" {
      n24 = call-poly "Variant to Data.vi"("Variant"=w85) -> ("Path"=w84:path)  [unwired: 8 in]
      n25 = Format Into String(format string=": %s", initial string=w88, error in=w87, w84) -> (resulting string=w83:string, error out=w82:errorcluster)
    }
    frame "Available Gate Names" {
      n26 = call "AlliGator Settings Storage.vi"("AlliGator Settings List"=AlliGator_Settings_List."Data Information:Available Channel Names", "Error In"=w94) -> ("Variant Data out"=w92:variant)  [unwired: 8 in, 1 out]
      n27 = call-poly "Variant to Data.vi"("Variant"=w92) -> ("String Array"=w89:string[])  [unwired: 8 in]
      n28 = Empty Array?(array=w89) -> (empty?=w91:bool)
      n29 = case shown="False" w91 {
        tunnel: [w98 "Gate" ("input 1")] -> w90
        tunnel: w89 -> [w100 _]
        frame False {
          n30 = call "Concatenate String Array.vi"("Separator (TAB)"=", ", "String Array"=w100) -> ("Formatted String"=w98:string)  [unwired: 9 in]
        }
        frame True {
        }
      }
      n31 = Format Into String(format string="Available Gate Names: %s", w90) -> (resulting string=w96:string, error out=w95:errorcluster)  [unwired: 2 in]
    }
    frame "Background Definition Range" {
      n32 = Variant To Data(error in=w103, type=T3 {"Min Gate"=0.0, "Max Gate"=8e-10} ("Background Definition Range"), Variant=w110) -> (data=w108:T3, error out=w102:errorcluster)
      n33 = Unbundle By Name(w108) -> ("Min Gate"=w107:dbl[unit], "Max Gate"=w106:dbl[unit])
      n34 = node(w106) -> (w104:dbl)
      n35 = node(w107) -> (w105:dbl)
      n36 = Format Into String(format string=": Min Gate: %#g ps, Max Gate: %#g ps", initial string=w114, error in=w102, w105, w104) -> (resulting string=w112:string, error out=w111:errorcluster)
    }
    frame "Average Lifetime Options" {
      n37 = call "Variant to Formatted String v2.vi"("error in (no error)"=w117, "Anything"=w118) -> ("error out"=w115:errorcluster, "String"=w116:string)  [unwired: 8 in]
    }
    frame "Backup Calibration Type" {
      n38 = Variant To Data(error in=w120, type=T4."Single Calibration" ("Backup Calibration"), Variant=w123) -> (data=w121:T4, error out=w119:errorcluster)
      n39 = Format Into String(format string=": %s", initial string=w127, error in=w119, w121) -> (resulting string=w125:string, error out=w124:errorcluster)
    }
    frame "Baseline Subtraction Method" {
      n40 = Variant To Data(error in=w129, type=AlliGator_Baseline_Subtraction_Method."Mean" ("Baseline Subtraction Method"), Variant=w132) -> (data=w131:T5, error out=w128:errorcluster)
      n41 = Format Into String(format string=": %s", initial string=w136, error in=w128, w131) -> (resulting string=w134:string, error out=w133:errorcluster)
    }
    frame "Calibration Type" {
      n42 = Variant To Data(error in=w139, type=Phasor_Calibration_Type."None" ("Calibration Type"), Variant=w141) -> (data=w140:T6, error out=w138:errorcluster)
      n43 = Format Into String(format string=": %s", initial string=w145, error in=w138, w140) -> (resulting string=w143:string, error out=w142:errorcluster)
    }
    frame "Calibration Map Algorithm" {
      n44 = Variant To Data(error in=w148, type=AlliGator_Calibration_Map_Algorithm."Min Distance" ("Calibration Map Algorithm"), Variant=w150) -> (data=w149:T7, error out=w147:errorcluster)
      n45 = Format Into String(format string=": %s", initial string=w154, error in=w147, w149) -> (resulting string=w152:string, error out=w151:errorcluster)
    }
    frame "Decay & IRF Parameters" {
      n46 = Variant To Data(error in=w160, type=T8 {"Lifetime"=0.0, "IRF Offset"=0.0, "IRF Period"=0.0, "Normalized Decays"=FALSE, "IRF Model"=enum."Dirac", "IRF Parameter 1"=0.0} ("Phasor Explorer Decay & IRF Parameters"), Variant=w161) -> (data=w159:T8, error out=w158:errorcluster)
      n47 = call "Variant to Formatted String v2.vi"("error in (no error)"=w158, "Anything"=w159) -> ("error out"=w156:errorcluster, "String"=w157:string)  [unwired: 8 in]
    }
    frame "Decay Analysis Parameters", "Decay Shift Parameters" {
      n48 = Variant To Data(error in=w164, type=T10 {"Type"=enum."Default", "Shift"=0.0, "Threshold"=0.0, "Rotate"=FALSE} ("Decay Shift Parameters"), Variant=w172) -> (data=w171:T10, error out=w163:errorcluster)
      n49 = Unbundle(w171) -> ("Type"=w169:T1, "Shift"=w168:dbl[unit], "Threshold"=w166:dbl, "Rotate"=w165:bool)
      n50 = case shown="\"Default\"" w169 {
        tunnel: w168 -> [w181 w189 _ _]
        tunnel: [w179 w187 w193 _] -> w167
        tunnel: w166 -> [_ _ w192 _]
        tunnel: w165 -> [_ w186 _ _]
        tunnel: w163 -> [w178 w184 w191 w195]
        tunnel: [w177 w183 w190 w195] -> w162
        frame "CFD" {
          n51 = node(w181) -> (w180:dbl)
          n52 = Format Into String(format string="\nShift: %#g ns", error in=w178, w180) -> (resulting string=w179:string, error out=w177:errorcluster)  [unwired: 1 in]
        }
        frame "Default" {
          n53 = node(w189) -> (w188:dbl)
          n54 = Format Into String(format string="\nShift: %#g ns\nRotate: %s", error in=w184, w188, w186) -> (resulting string=w187:string, error out=w183:errorcluster)  [unwired: 1 in]
        }
        frame "Threshold" {
          n55 = Format Into String(format string="\nValue: %#g", error in=w191, w192) -> (resulting string=w193:string, error out=w190:errorcluster)  [unwired: 1 in]
        }
        frame "Cross-Correlation" {
        }
      }
      n56 = Format Into String(format string="\nType: %s%s", initial string=w176, error in=w162, w169, w167) -> (resulting string=w174:string, error out=w173:errorcluster)
    }
    frame "Decay Graph Color Array" {
      n57 = Variant To Data(error in=w202, type=u32[] [0, 1, 2, 3, 4, 5, 6, 7, 8, 10, 11] ("Displayed Fit Parameters"), Variant=w203) -> (data=w197:u32[], error out=w198:errorcluster)
      n58 = Empty Array?(array=w197) -> (empty?=w196:bool)
      n59 = case shown="True" w196 {
        tunnel: w197 -> [_ w210]
        tunnel: w200 -> [_ w209]
        tunnel: [_ w205] -> w199
        frame False {
        }
        frame True {
          n60 = Concatenate Strings(w209, ":" ("string")) -> (w207:string)
          n61 = for {
            tunnel: w210 -> [w214] mode=indexing
            shift-right: [w211] -> w208
            shift-left: w207 -> [w213]
            n62 = Format Into String(format string="\\n%d", initial string=w213, w214) -> (resulting string=w211:string)  [unwired: 1 in, 1 out]
          }
          n63 = Concatenate Strings(w208, "\r\n") -> (w205:string)
        }
      }
    }
    frame "Define Gates to" {
      n64 = Variant To Data(error in=w219, type=AlliGator_Define_Gates_to."Skip" ("Define Gates to"), Variant=w220) -> (data=w216:T11, error out=w218:errorcluster)
      n65 = case shown="\"Skip\", Default" w216 {
        tunnel: ["Skip" ("input 1") "Keep" ("input 1")] -> w215
        frame "Skip", Default {
        }
        frame "Keep" {
        }
      }
      n66 = Format Into String(format string="Using Gates to %s option", error in=w218, w215) -> (resulting string=w222:string, error out=w221:errorcluster)  [unwired: 1 in]
    }
    frame "Define Shortest Lifetime as" {
      n67 = Variant To Data(error in=w230, type=enum32{"Item 0", "Item 1"}."Item 0" ("Define Gates to"), Variant=w231) -> (data=w227:enum32{"Item 0", "Item 1"}, error out=w229:errorcluster)
      n68 = case shown="\"Item 1\"" w227 {
        tunnel: ["Reference 1" ("input 1") "Reference 2" ("input 1")] -> w226
        frame "Item 0", Default {
        }
        frame "Item 1" {
        }
      }
      n69 = Format Into String(format string="Defining Shortest Lifetime as %s", error in=w229, w226) -> (resulting string=w233:string, error out=w232:errorcluster)  [unwired: 1 in]
    }
    frame "Display Parameters" {
      n70 = Variant To Data(error in=w242, type=T12 {"# Points"=1, "Ramp Type"=enum."Linear", "Type of Series"=enum."1-Exp Decays", "Min tau"=0.0, "Max tau"=0.0, "Include 0"=FALSE, "Include Infinity"=FALSE} ("Phasor Explorer Display Parameters"), Variant=w243) -> (data=w241:T12, error out=w240:errorcluster)
      n71 = call "Variant to Formatted String v2.vi"("error in (no error)"=w240, "Anything"=w241) -> ("error out"=w238:errorcluster, "String"=w239:string)  [unwired: 8 in]
    }
    frame "Displayed Fit Parameters" {
      w249 = T46[] [] items=["Offset", "Baseline", "A_1", "tau_1", "A_2", "tau_2", "<tau>_a", "f1_a", "f2_a", "<tau>_i", "f1_i", "f2_i", "-", "R^2", "Chi^2"] ("Displayed Fit Parameters")
      n72 = Variant To Data(error in=w250, type=w249, Variant=w251) -> (data=w245:T46[], error out=w247:errorcluster)
      n73 = Empty Array?(array=w245) -> (empty?=w244:bool)
      n74 = case shown="False" w244 {
        tunnel: w245 -> [w257 _]
        tunnel: [w252 _] -> w248
        tunnel: w246 -> [w255 _]
        frame False {
          n75 = Concatenate Strings("\r\n", w255, ":" ("string")) -> (w254:string)
          n76 = for {
            tunnel: w257 -> [w261] mode=indexing
            shift-right: [w258] -> w252
            shift-left: w254 -> [w260]
            n77 = Format Into String(format string="\\n%s", initial string=w260, w261) -> (resulting string=w258:string)  [unwired: 1 in, 1 out]
          }
        }
        frame True {
        }
      }
    }
    frame "Exported Gate Image Settings", "Fit Options", "Histogram Options", "Image Binning Options", "Image Smoothing Options", "Phasor Plot Graphics Options", "Phasor Plot Smoothing Options" {
      n78 = call "Variant to Formatted String v2.vi"("error in (no error)"=w264, "Anything"=w265) -> ("error out"=w262:errorcluster, "String"=w263:string)  [unwired: 8 in]
    }
    frame "Fit Parameter Constraints" {
      n79 = Variant To Data(error in=w271, type=T14[] [{"Fit Parameter"=enum."A_1", "Min Value"=0.0, "Max Value"=inf, "Global"=FALSE, "Used"=FALSE}, {"Fit Parameter"=enum."tau_1", "Min Value"=0.05, "Max Value"=inf, "Global"=TRUE, "Used"=FALSE}, {"Fit Parameter"=enum."A_2", "Min Value"=0.0, "Max Value"=inf, "Global"=FALSE, "Used"=FALSE}, {"Fit Parameter"=enum."tau_2", "Min Value"=0.05, "Max Value"=inf, "Global"=TRUE, "Used"=FALSE}] ("Fit Parameter Constraints"), Variant=w272) -> (data=w267:T14[], error out=w268:errorcluster)
      n80 = Empty Array?(array=w267) -> (empty?=w266:bool)
      n81 = case shown="False" w266 {
        tunnel: [w280 _] -> w274
        tunnel: [w279 w288] -> w273
        tunnel: w269 -> [w276 _]
        tunnel: w268 -> [w278 w288]
        tunnel: w267 -> [w277 _]
        frame False {
          n82 = for {
            tunnel: w277 -> [w286] mode=indexing
            shift-right: [w284] -> w280
            shift-left: "" -> [w283]
            tunnel: w276 -> [_]
            shift-right: [w287] -> w279
            shift-left: w278 -> [w285]
            w281 = "\r\n"
            n83 = call "Variant to Formatted String v2.vi"("error in (no error)"=w285, "Anything"=w286) -> ("error out"=w287:errorcluster, "String"=w282:string)  [unwired: 8 in]
            n84 = Concatenate Strings(w283, w281, w282, w281) -> (w284:string)
          }
        }
        frame True {
        }
      }
    }
    frame "Channel Name" {
      n85 = call "AlliGator Settings Storage.vi"("AlliGator Settings List"=AlliGator_Settings_List."Data Information:Available Channel Names", "Error In"=w296) -> ("Variant Data out"=w294:variant)  [unwired: 8 in, 1 out]
      n86 = call-poly "Variant to Data.vi"("Variant"=w297) -> ("U16 Value"=w293:u16)  [unwired: 8 in]
      n87 = call-poly "Variant to Data.vi"("Variant"=w294) -> ("String Array"=w292:string[])  [unwired: 8 in]
      n88 = Empty Array?(array=w292) -> (empty?=w291:bool)
      n89 = Index Array(array=w292, index=w293) -> (element=w289:string)
      n90 = case shown="False" w291 {
        tunnel: [w301 "Gate" ("input 1")] -> w290
        tunnel: w289 -> [w301 _]
        frame False {
        }
        frame True {
        }
      }
      n91 = Format Into String(format string="Channel Name: %s", w290) -> (resulting string=w299:string, error out=w298:errorcluster)  [unwired: 2 in]
    }
    frame "Gate Parameters" {
      n92 = Variant To Data(error in=w308, type=T16 {"First Gate Start"=0.0, "Use Gate Center"=FALSE, "Gate Width"=0.0, "Gate Step"=0.0, "# Gates"=1.0, "Gate Type"=enum."Square", "Edge Width"=0.0, "Top Slope"=0.0, "Reversed Sawtooth?"=FALSE, "Analytical Computation"=FALSE, "Integration"=enum."Item 0", "Tolerance"=1.0, "# Steps"=1.0, "Type of User-defined Function"=enum."Gate", "Use Gate Step"=FALSE} ("Phasor Explorer Gate Parameters"), Variant=w309) -> (data=w306:T16, error out=w305:errorcluster)
      n93 = call "Variant to Formatted String v2.vi"("error in (no error)"=w305, "Anything"=w306) -> ("error out"=w303:errorcluster, "String"=w304:string)  [unwired: 8 in]
    }
    frame "Channel Arithmetic" {
      n94 = Variant To Data(error in=w317, type=AlliGator_Gate_Arithmetic."None" ("Gate Arithmetic"), Variant=w318) -> (data=w316:T19, error out=w315:errorcluster)
      n95 = Format Into String(format string=": %s", initial string=w314, error in=w315, w316) -> (resulting string=w311:string, error out=w312:errorcluster)
    }
    frame "Gates to Keep" {
      n96 = Variant To Data(error in=w320, type=T20 {"First"=0, "Last"=0} ("Decay Points to Skip"), Variant=w325) -> (data=w324:T20, error out=w319:errorcluster)
      n97 = Unbundle By Name(w324) -> ("First"=w323:u32, "Last"=w322:u32)
      n98 = Format Into String(format string=": First: %d, Last: %d", initial string=w329, error in=w319, w323, w322) -> (resulting string=w327:string, error out=w326:errorcluster)
    }
    frame "MLE Baseline Offset Type" {
      n99 = Variant To Data(error in=w333, type=MLE_Baseline_Offset_Type."Absolute" ("MLE Baseline Offset Type"), Variant=w334) -> (data=w330:T21, error out=w332:errorcluster)
      n100 = Format Into String(format string=": %s", initial string=w338, error in=w332, w330) -> (resulting string=w336:string, error out=w335:errorcluster)
    }
    frame "Gates to Skip" {
      n101 = Variant To Data(error in=w340, type=T22 {"Start"=0, "End"=0} ("Decay Points to Skip"), Variant=w345) -> (data=w344:T22, error out=w339:errorcluster)
      n102 = Unbundle By Name(w344) -> ("Start"=w343:u32, "End"=w342:u32)
      n103 = Format Into String(format string=": from Start: %d, from End: %d", initial string=w349, error in=w339, w343, w342) -> (resulting string=w347:string, error out=w346:errorcluster)
    }
    frame "Hot Pixel Removal" {
      n104 = Variant To Data(error in=w352, type=T23 {"Remove Screamers"=FALSE, "Delta"=0.0, "Equalize Histogram"=FALSE, "Percentile"=0.0, "Hot Pixel Mask Image"=path "", "Use Hot Pixel Mask"=FALSE} ("Image Display Options"), Variant=w354) -> (data=w353:T23, error out=w351:errorcluster)
      n105 = call "AlliGator Hot Pixel Removal Options String.vi"("error in (no error)"=w351, "Image Display Options"=w353) -> ("error out"=w355:errorcluster, "String out"=w356:string)  [unwired: 8 in]
    }
    frame "Phasor Ratio Type" {
      n106 = Variant To Data(error in=w361, type=Phasor_Ratio_Type."Intensity-weighted" ("Phasor Ratio Type"), Variant=w362) -> (data=w358:T24, error out=w360:errorcluster)
      n107 = case shown="\"Amplitude-weighted\"" w358 {
        tunnel: ["Intensity" ("input 1") "Amplitude" ("input 1")] -> w357
        frame "Intensity-weighted", Default {
        }
        frame "Amplitude-weighted" {
        }
      }
      n108 = Format Into String(format string=": %s-weighted", initial string=w366, error in=w360, w357) -> (resulting string=w364:string, error out=w363:errorcluster)
    }
    frame "Guess Parameter Names" {
      w372 = T15[] [] items=["Offset", "Baseline", "A_1", "tau_1", "A_2", "tau_2"] ("Array")
      w369 = ":\n"
      n109 = Variant To Data(error in=w374, type=w372, Variant=w375) -> (data=w371:T15[], error out=w373:errorcluster)
      n110 = for {
        tunnel: w371 -> [w381] mode=indexing
        tunnel: [w380] -> w370 mode=indexing
        n111 = Format Into String(w381) -> (resulting string=w380:string)  [unwired: 3 in, 1 out]
      }
      n112 = call "Concatenate String Array.vi"("Separator (TAB)"="        ", "String Array"=w370) -> ("Formatted String"=w378:string)  [unwired: 9 in]
      n113 = Concatenate Strings(w369, w377, w369, w378) -> (w376:string)
    }
    frame "Guess Parameters" {
      w382 = ":\n"
      n114 = call-poly "Variant to Data.vi"("Variant"=w389) -> ("Value"=w386:dbl[])  [unwired: 8 in]
      n115 = Array To Spreadsheet String(delimiter (Tab)="        " ("Separator (TAB)"), array=w386, 3:"%#g" ("format string")) -> (spreadsheet string=w383:string)
      n116 = Concatenate Strings(w382, w388, w382, w383) -> (w387:string)
    }
    frame "High Count Pixels Rejection Options" {
      n117 = Variant To Data(error in=w393, type=T25 {"Background High Threshold Factor"=0.0, "Fixed High Background Threshold"=17000.0, "Reject High Count Pixels"=FALSE, "High Percentile"=100.0} ("Low Count Pixels Rejection Options 2"), Variant=w399) -> (data=w398:T25, error out=w392:errorcluster)
      n118 = Unbundle By Name(w398) -> ("Reject High Count Pixels"=w396:bool, "Background High Threshold Factor"=w395:dbl, "Fixed High Background Threshold"=w394:dbl, "High Percentile"=w391:dbl)
      n119 = Format Into String(format string=":\nReject High Count Pixels: %s\nPeak Threshold x Factor: %#g\nFixed Peak Threshold: %#g\n\nHigh Percentile: %#g", initial string=w403, error in=w392, w396, w395, w394, w391) -> (resulting string=w401:string, error out=w400:errorcluster)
    }
    frame "IRF Analysis Parameters" {
      n120 = Variant To Data(error in=w405, type=T10 {"Type"=enum."Default", "Shift"=0.0, "Threshold"=0.0, "Rotate"=FALSE} ("IRF Analysis Method"), Variant=w414) -> (data=w413:T10, error out=w404:errorcluster)
      n121 = Unbundle By Name(w413) -> ("Type"=w407:T1, "Shift"=w412:dbl[unit], "Threshold"=w411:dbl)
      n122 = property on="Type" class="Enum (strict)"() -> ("Strings []"=w406:string[])  [unwired: 2 in, 2 out]
      n123 = Index Array(array=w406, index=w407) -> (element=w409:string)
      n124 = node(w412) -> (w408:dbl)
      n125 = case shown="\"CFD\"" w407 {
        tunnel: w417 -> [w424 w431 w437]
        tunnel: w404 -> [w423 w430 w436]
        tunnel: [w422 w429 w435] -> w416
        tunnel: [w421 w428 w434] -> w415
        tunnel: w411 -> [_ w425 _]
        tunnel: w409 -> [w420 w427 w433]
        tunnel: w408 -> [w419 _ _]
        frame "CFD" {
          n126 = Format Into String(format string=": Type: %s, Shift %#g ns", initial string=w424, error in=w423, w420, w419) -> (resulting string=w422:string, error out=w421:errorcluster)
        }
        frame "Threshold" {
          n127 = Format Into String(format string=": Type: %s, Threshold %#g", initial string=w431, error in=w430, w427, w425) -> (resulting string=w429:string, error out=w428:errorcluster)
        }
        frame "Default", Default {
          n128 = Format Into String(format string=": Type: %s", initial string=w437, error in=w436, w433) -> (resulting string=w435:string, error out=w434:errorcluster)
        }
      }
    }
    frame "IRF Extraction Options" {
      n129 = Variant To Data(error in=w453, type=T26 {"Time Constant for IRF Extraction"=4.08e-09, "IRF Order"=132, "Fourier Series Smoothing"=enum."Fejer Summation", "Noise Threshold"=0.1, "Smoothing Width"=0.1, "Fourier Series Truncation"=enum."Automatic", "Truncation Order"=0, "Save Power Spectrum"=FALSE, "Smoothing"=FALSE, "Smoothing Parameter"=0.0, "Smoothing Order"=1, "Method"=enum."Direct"} ("IRF Extraction Options"), Variant=w456) -> (data=w455:T26, error out=w452:errorcluster)
      n130 = Unbundle By Name(w455) -> ("Time Constant for IRF Extraction"=w450:dbl[unit], "Fourier Series Smoothing"=w449:T27, "Noise Threshold"=w448:dbl, "Smoothing Width"=w447:dbl, "Fourier Series Truncation"=w446:T28, "Truncation Order"=w445:i32, "Save Power Spectrum"=w444:bool, "Smoothing"=w443:bool, "Smoothing Parameter"=w442:dbl, "Smoothing Order"=w441:u32, "Method"=w439:T29)
      n131 = node(w450) -> (w440:dbl)
      n132 = Format Into String(w439) -> (resulting string=w438:string)  [unwired: 3 in, 1 out]
      n133 = Format Into String(format string=":\n    Time Constant: %#g ns\n    Smoothing Algorithm: %s\n    Noise Threshold: %#g\n    Smoothing Width: %#g\n    Fourier Series Truncation: %s\n    Fourier Truncation Order: %d\n    Save Power Spectrum: %s\nSmoothing: %s\nSmoothing Parameter: %#g\nSmoothing Order: %d\nMethods: %s", initial string=w459, error in=w452, w440, w449, w448, w447, w446, w445, w444, w443, w442, w441, w438) -> (resulting string=w458:string, error out=w457:errorcluster)
    }
    frame "IRF Optimization Options" {
      n134 = call "Variant to Formatted String v2.vi"("error in (no error)"=w462, "Anything"=w463) -> ("error out"=w461:errorcluster, "String"=w460:string)  [unwired: 8 in]
    }
    frame "IRF Time Constants", "Lifetime Map Active" {
      # "Silent controls"
    }
    frame "Kernel Type" {
      n135 = Variant To Data(error in=w466, type=Kernel_Type."Uniform" ("Kernel Type"), Variant=w469) -> (data=w468:T30, error out=w465:errorcluster)
      n136 = Format Into String(format string=": %s", initial string=w473, error in=w465, w468) -> (resulting string=w471:string, error out=w470:errorcluster)
    }
    frame "Low Count Pixels Rejection Options" {
      n137 = Variant To Data(error in=w475, type=T31 {"Background Low Threshold Factor"=0.0, "Fixed Low Background Threshold"=17000.0, "Reject Low Count Pixels"=FALSE, "Low Percentile"=0.0} ("Low Count Pixels Rejection Options"), Variant=w482) -> (data=w481:T31, error out=w474:errorcluster)
      n138 = Unbundle By Name(w481) -> ("Reject Low Count Pixels"=w479:bool, "Background Low Threshold Factor"=w478:dbl, "Fixed Low Background Threshold"=w477:dbl, "Low Percentile"=w476:dbl)
      n139 = Format Into String(format string=":\nReject Low Count Pixels: %s\nBackground Threshold x Factor: %#g\nFixed Background Threshold: %#g\n\nLow Percentile: %#g", initial string=w486, error in=w474, w479, w478, w477, w476) -> (resulting string=w484:string, error out=w483:errorcluster)
    }
    frame "Operation Order" {
      n140 = call "AlliGator Settings Storage.vi"("AlliGator Settings List"=AlliGator_Settings_List."GUI:Visible Settings Tab", "Error In"=w488) -> ("Error Out"=w489:errorcluster, "Variant Data out"=w490:variant)  [unwired: 8 in]
      n141 = call-poly "Variant to Data.vi"("Variant"=w490) -> ("String Array"=w493:string[])  [unwired: 8 in]
      n142 = call "Concatenate String Array.vi"("Separator (TAB)"=", ", "String Array"=w493) -> ("Formatted String"=w491:string)  [unwired: 9 in]
      n143 = Format Into String(format string=": %s", initial string=w495, error in=w489, w491) -> (resulting string=w496:string, error out=w497:errorcluster)
    }
    frame "Operations Order" {
      n144 = call-poly "Variant to Data.vi"("Variant"=w506) -> ("String Array"=w504:string[])  [unwired: 8 in]
      n145 = call "Concatenate String Array.vi"("Separator (TAB)"=", ", "String Array"=w504) -> ("Formatted String"=w503:string)  [unwired: 9 in]
      n146 = Format Into String(format string=": %s", initial string=w502, error in=w498, w503) -> (resulting string=w499:string, error out=w505:errorcluster)
    }
    frame "Phasor Parameters" {
      n147 = Variant To Data(error in=w512, type=T32 {"Harmonic Frequency"=0.0, "Use f* = 1/D Frequency"=FALSE, "Calibrated Phasor"=FALSE, "Calibration Lifetime"=1e-09, "Phasor Calculation"=enum."Direct Sum", "SEPL Type"=enum."UC", "# Gates"=1.0, "Square Gate Width"=1e-09, "Show Ticks"=FALSE} ("Phasor Explorer Phasor Parameters"), Variant=w513) -> (data=w511:T32, error out=w510:errorcluster)
      n148 = call "Variant to Formatted String v2.vi"("error in (no error)"=w510, "Anything"=w511) -> ("error out"=w508:errorcluster, "String"=w509:string)  [unwired: 8 in]
    }
    frame "Phasor Plot Display Range" {
      n149 = Variant To Data(error in=w515, type=cluster{u16, u16} {0, 100} ("Phasor Plot Display Range"), Variant=w520) -> (data=w519:cluster{u16, u16}, error out=w514:errorcluster)
      n150 = Unbundle(w519) -> (w518:u16, w517:u16)
      n151 = Format Into String(format string=": Min: %d, Max: %d", initial string=w524, error in=w514, w518, w517) -> (resulting string=w522:string, error out=w521:errorcluster)
    }
    frame "Phasor Plot Size" {
      n152 = Variant To Data(error in=w526, type=T35 {"H"=512, "V"=512, "Margin"=0.2} ("Phasor Plot Size"), Variant=w532) -> (data=w531:T35, error out=w525:errorcluster)
      n153 = Unbundle By Name(w531) -> ("H"=w530:i32, "V"=w529:i32, "Margin"=w527:dbl)
      n154 = Format Into String(format string=": H: %d, V: %d, Margin: %#g", initial string=w536, error in=w525, w530, w529, w527) -> (resulting string=w534:string, error out=w533:errorcluster)
    }
    frame "Phasor Ratio Color Map Type" {
      n155 = Variant To Data(error in=w544, type=T36."Interpolate Reference Colors" ("Phasor Ratio Color Map Type"), Variant=w545) -> (data=w537:T36, error out=w543:errorcluster)
      n156 = Format Into String(format string=": %s", initial string=w540, error in=w543, w537) -> (resulting string=w541:string, error out=w542:errorcluster)
    }
    frame "Phasor Ratio Color-Coded Quantity" {
      n157 = Variant To Data(error in=w549, type=AlliGator_Phasor_Ratio_Color-Coded_Quantity."Phasor Ratio (f1 or a1)" ("Displayed Quantity"), Variant=w551) -> (data=w547:T37, error out=w548:errorcluster)
      n158 = Format Into String(format string="%s: %s", error in=w548, w546, w547) -> (resulting string=w553:string, error out=w552:errorcluster)  [unwired: 1 in]
    }
    frame "Phasor Ratio Display Range" {
      n159 = Variant To Data(error in=w557, type=cluster{"Min":dbl, "Max":dbl} {"Min"=0.0, "Max"=1.0} ("Phasor Ratio Display Range"), Variant=w561) -> (data=w560:cluster{"Min":dbl, "Max":dbl}, error out=w556:errorcluster)
      n160 = Unbundle By Name(w560) -> ("Min"=w559:dbl, "Max"=w558:dbl)
      n161 = Format Into String(format string=": Min: %#g, Max: %#g", initial string=w565, error in=w556, w559, w558) -> (resulting string=w563:string, error out=w562:errorcluster)
    }
    frame "Phasor Ratio Reference Colors" {
      n162 = Variant To Data(error in=w567, type=T38 {"Reference 1"=3381759, "Reference 2"=3381759, "Boundary"=3381759} ("Phasor Ratio Reference Colors"), Variant=w573) -> (data=w572:T38, error out=w566:errorcluster)
      n163 = Unbundle By Name(w572) -> ("Reference 1"=w571:u32, "Reference 2"=w570:u32, "Boundary"=w569:u32)
      n164 = Format Into String(format string=":\nReference 1: %d\nReference 2: %d\nBoundary: %d", initial string=w577, error in=w566, w571, w570, w569) -> (resulting string=w575:string, error out=w574:errorcluster)
    }
    frame "Pseudo UC Add'l Parameters" {
      n165 = Variant To Data(error in=w579, type=T39 {"Laser Period"=1e-09, "Decay Offset"=1e-09} ("Pseudo UC Add'l Parameters"), Variant=w587) -> (data=w586:T39, error out=w578:errorcluster)
      n166 = Unbundle By Name(w586) -> ("Laser Period"=w584:dbl[unit], "Decay Offset"=w585:dbl[unit])
      n167 = node(w585) -> (w582:dbl)
      n168 = node(w584) -> (w580:dbl)
      n169 = Format Into String(format string=":\nLaser Period: %#g ns\nDecay Offset: %#g ns", initial string=w590, error in=w578, w580, w582) -> (resulting string=w589:string, error out=w588:errorcluster)
    }
    frame "Python Settings" {
      # "\"Python Settings\""
      n170 = Variant To Data(error in=w595, type=T40 {"Python Version"="", "Use PATH definition"=FALSE, "Python.exe Path"=path "", "Include Example Plugins"=FALSE} ("Python Settings"), Variant=w598) -> (data=w597:T40, error out=w594:errorcluster)
      n171 = Unbundle By Name(w597) -> ("Python Version"=w592:string, "Python.exe Path"=w591:path)
      n172 = Format Into String(format string=":\nVersion %s\nPyton.exe Path: %s", initial string=w601, error in=w594, w592, w591) -> (resulting string=w600:string, error out=w599:errorcluster)
    }
    frame "Reference Curve" {
      n173 = Variant To Data(error in=w604, type=enum32{"UC", "Pseudo UC"}."UC" ("Reference Circle"), Variant=w607) -> (data=w602:enum32{"UC", "Pseudo UC"}, error out=w603:errorcluster)
      n174 = Format Into String(format string=": %s", initial string=w610, error in=w603, w602) -> (resulting string=w609:string, error out=w608:errorcluster)
    }
    frame "Saved Displayed Image File Format" {
      n175 = Variant To Data(error in=w612, type=Image_Save_File_Format."PNG" ("Saved Image File Format"), Variant=w615) -> (data=w614:T41, error out=w611:errorcluster)
      n176 = Format Into String(format string=": %s", initial string=w619, error in=w611, w614) -> (resulting string=w617:string, error out=w616:errorcluster)
    }
    frame "Saved Image File Format" {
      n177 = Variant To Data(error in=w627, type=Image_Save_File_Format."PNG" ("Saved Image File Format"), Variant=w628) -> (data=w623:T41, error out=w621:errorcluster)
      n178 = Format Into String(format string=": %s", initial string=w625, error in=w621, w623) -> (resulting string=w622:string, error out=w620:errorcluster)
    }
    frame "Square Pulse Options" {
      n179 = Variant To Data(error in=w633, type=T42 {"Method"=enum."Mode", "# Bins"=0, "Threshold %"=0.0, "Center on Midpoint"=FALSE, "Smoothen Plot"=FALSE} ("IRF Analysis Method"), Variant=w635) -> (data=w631:T42, error out=w632:errorcluster)
      n180 = call "Square Pulse Options String.vi"("Error In"=w632, "Square Pulse Options"=w631) -> ("Error Out"=w629:errorcluster, "Option String"=w630:string)  [unwired: 8 in]
    }
    frame "Type" {
      n181 = Variant To Data(error in=w637, type=XY_Graph_Plot_Shift_Method."Default" ("IRF Analysis Method"), Variant=w640) -> (data=w639:T1, error out=w636:errorcluster)
      n182 = Format Into String(format string="Decay Shift Type: %s", error in=w636, w639) -> (resulting string=w642:string, error out=w641:errorcluster)  [unwired: 1 in]
    }
    frame "User-defined Gate", "User-defined IRF" {
      n183 = Variant To Data(error in=w656, type=T44 {"X Array"=[], "Y Array"=[]} ("Plot"), Variant=w655) -> (data=w653:T44, error out=w645:errorcluster)
      n184 = Unbundle By Name(w653) -> ("X Array"=w652:dbl[])
      n185 = Array Size(array=w652) -> (size(s)=w651:i32)
      n186 = case shown="0" w651 {
        selector: w651 -> [_ w661]
        tunnel: [" undefined..." ("input 1") w663] -> w646
        tunnel: w645 -> [w657 w660]
        tunnel: [w657 w659] -> w644
        frame 0 {
        }
        frame 1, Default {
          n187 = Format Into String(format string=": %d points", error in=w660, w661) -> (resulting string=w663:string, error out=w659:errorcluster)  [unwired: 1 in]
        }
      }
      n188 = Format Into String(format string="%s", initial string=w648, error in=w644, w646) -> (resulting string=w650:string, error out=w649:errorcluster)
    }
    frame "Wavelet Analysis Options" {
      n189 = Variant To Data(error in=w671, type=T45 {"Wavelet"=enum."db02", "Option for Approximate Coefficients"=enum."None", "# Levels"=0, "Threshold Settings"={"Thresholding Rule"=enum."Universal", "Rescaling Method"=enum."Single level", "Soft Threshold?"=TRUE}, "Wavelet Transform Type"=enum."Discrete"} ("IRF Analysis Method"), Variant=w676) -> (data=w675:T45, error out=w670:errorcluster)
      n190 = Unbundle By Name(w675) -> ("Wavelet Transform Type"=w673:enum16{"Discrete", "Undecimated"}, "Wavelet"=w669:T47, "Option for Approximate Coefficients"=w668:enum16{"None", "Threshold", "Detrend"}, "# Levels"=w667:i32, "Threshold Settings.Thresholding Rule"=w666:enum16{"SURE", "Hybrid", "Universal", "Minimax"}, "Threshold Settings.Rescaling Method"=w665:enum16{"One", "Single level", "Multiple levels"}, "Threshold Settings.Soft Threshold?"=w664:bool)
      n191 = Format Into String(format string=":\n    Wavelet Transform Type: %s\n    Wavelet: %s\n    Option for Approximate Coefficients: %s\n    # Levels: %d\n    Thresholding Rule: %s\n     Rescaling Method: %s\n    Soft Threshold: %s", initial string=w679, error in=w670, w673, w669, w668, w667, w666, w665, w664) -> (resulting string=w678:string, error out=w677:errorcluster)
    }
    frame Default {
      n192 = call "Variant to Formatted String v2.vi"("error in (no error)"=w681, "Anything"=w680) -> ("error out"=w682:errorcluster, "String"=w683:string)  [unwired: 8 in]
    }
  }
  "error out" <- w4
  "Notebook String" <- w3
